vi "CTL_Calc_Level.vi"(5 "Drain IN":bool, 7 "Fill IN":bool, 9 "Level PV in":dbl, 10 "Max Fill Rate":dbl, 11 "Flow Rate %":dbl) -> (3 "PV Level Inch":dbl)   [LabVIEW 2024]
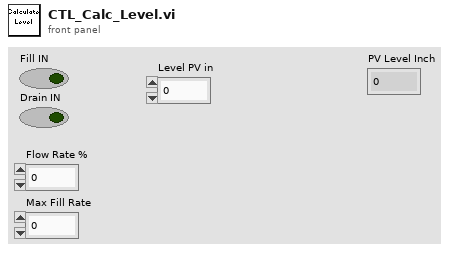
[diagram p1: front panel]
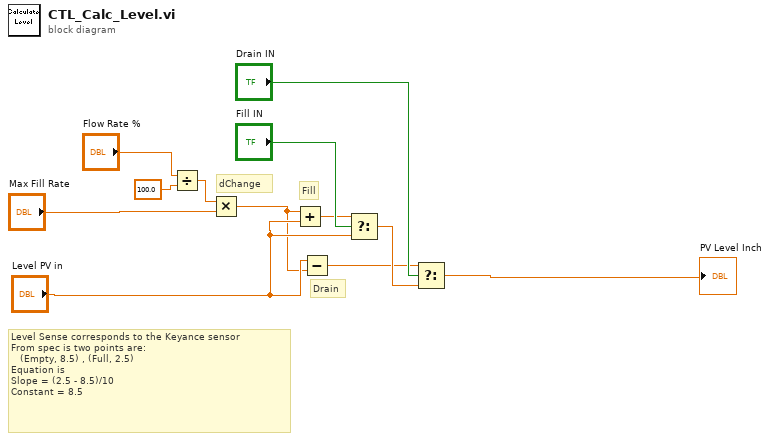
[diagram p0: block diagram]
diagram:
  # "Level Sense corresponds to the Keyance sensor\nFrom spec is two points are:\n   (Empty, 8.5) , (Full, 2.5)\nEquation is \nSlope = (2.5 - 8.5)/10\nConstant = 8.5"
  # "dChange"
  # "Drain"
  # "Fill"
  n1 = Divide(x="Flow Rate %", y=100.0) -> (x/y=w5:dbl)
  n2 = Multiply(x=w5, y="Max Fill Rate") -> (x*y=w6:dbl)
  n3 = Add(x=w6, y="Level PV in") -> (x+y=w1:dbl)
  n4 = Subtract(x="Level PV in", y=w6) -> (x-y=w2:dbl)
  n5 = Select(t=w1, s="Fill IN", f="Level PV in") -> (s? t:f=w3:dbl)
  n6 = Select(t=w2, s="Drain IN", f=w3) -> (s? t:f=→"PV Level Inch":dbl)
